vi "Crop2DMatrix.vi"(10 "Crop Pixels":u16=30, 11 "Data":dbl[][](array[numeric])) -> (3 "Cropped Data":dbl[][](array[numeric]))   [LabVIEW 2018]
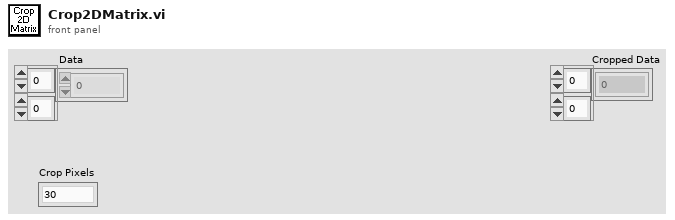
[diagram p1: front panel]
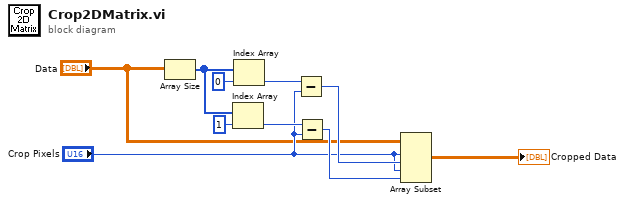
[diagram p0: block diagram]
diagram:
  n1 = Array Size(array="Data") -> (size(s)=w10:i32[])
  n2 = Index Array(array=w10, index=1) -> (element=w5:i32)
  n3 = Index Array(array=w10, index=0) -> (element=w7:i32)
  n4 = Subtract(x=w7, y="Crop Pixels") -> (x-y=w6:i32)
  n5 = Subtract(x=w5, y="Crop Pixels") -> (x-y=w4:i32)
  n6 = Array Subset(array="Data", index (row)="Crop Pixels", length (row)=w6, index (col)="Crop Pixels", length (col)=w4) -> (→"Cropped Data":dbl[][])
